vi "Build header single level.vi"(6 "Overvoltage":dbl, 7 "Recommended at 25C":bool, 8 "Add timestamp":bool=TRUE, 9 "MPPC Serial number":i32, 10 "ROB ID":i32, 11 "Scintillator ID":i32) -> (2 "Header":string)   [LabVIEW 2016]
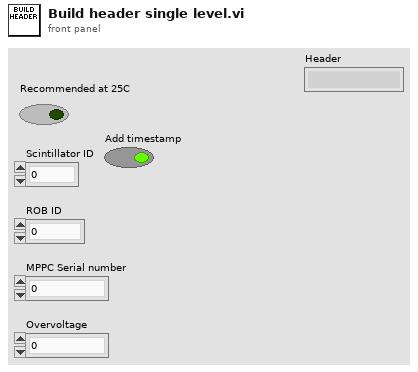
[diagram p1: front panel]
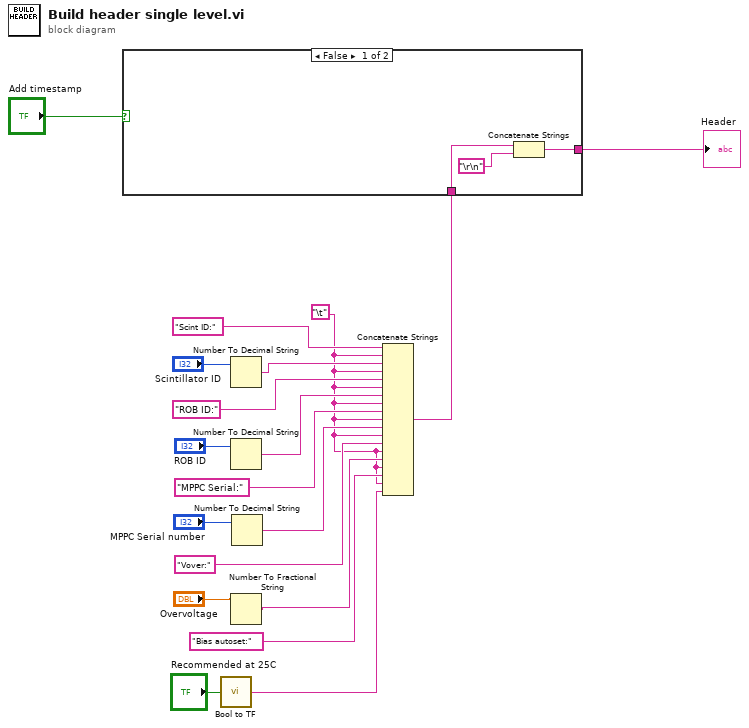
[diagram p0: block diagram]
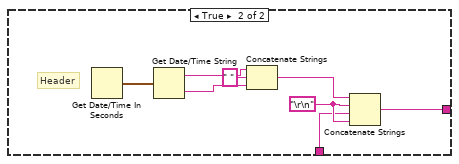
[diagram p2: hidden frame]
diagram:
  w2 = "\t"
  n1 = call "Bool to TF.vi"("Boolean"="Recommended at 25C") -> ("T/F"=w19:string)
  n2 = Number To Decimal String(number="Scintillator ID") -> (decimal integer string=w8:string)  [unwired: 1 in]
  n3 = Number To Decimal String(number="ROB ID") -> (decimal integer string=w10:string)  [unwired: 1 in]
  n4 = Number To Fractional String(number="Overvoltage") -> (F-format string=w16:string)  [unwired: 3 in]
  n5 = Number To Decimal String(number="MPPC Serial number") -> (decimal integer string=w12:string)  [unwired: 1 in]
  n6 = Concatenate Strings("Scint ID:", w2, w8, w2, "ROB ID:", w2, w10, w2, "MPPC Serial:", w2, w12, w2, "Vover:", w2, w16, w2, "Bias autoset:" ("string"), w2, w19) -> (w13:string)
  n7 = case shown="False" "Add timestamp" {
    tunnel: w13 -> [w22 w29]
    tunnel: [w20 w25] -> w3
    frame False {
      n8 = Concatenate Strings(w22, "\r\n") -> (w20:string)
    }
    frame True {
      w30 = "\r\n"
      # "Header"
      n9 = Get Date/Time In Seconds() -> (seconds since 1Jan1904=w26:timestamp)
      n10 = Get Date/Time String(seconds (now)=w26) -> (date string=w24:string, time string=w27:string)  [unwired: 2 in]
      n11 = Concatenate Strings(w24, " " ("string"), w27) -> (w28:string)
      n12 = Concatenate Strings(w28, w30, w29, w30) -> (w25:string)
    }
  }
  "Header" <- w3
